vi "Store Configuration Parameters.vi"(8 "error in (no error)":errorcluster, 10 "refnum":T1, 11 "Example Configuration Dialog in":refnum<class "Server Config.lvclass">) -> (0 "error out":errorcluster, 2 "refnum out":T1, 3 "Example Configuration Dialog out":refnum<class "Server Config.lvclass">)   [LabVIEW 2016, in "Server Controller.lvlib" / "Server Config.lvclass"]
uses:
  Server Config.lvclass
  <vilib>/Utility/config.llb/Config Data RefNum.ctl
  Server Config.lvclass/Server Config.ctl
  MAL-Framework/user.lib/Common Components/Msmt Configuration/Controller Configuration.lvclass
  <vilib>/Utility/config.llb/NI_LVConfig.lvlib
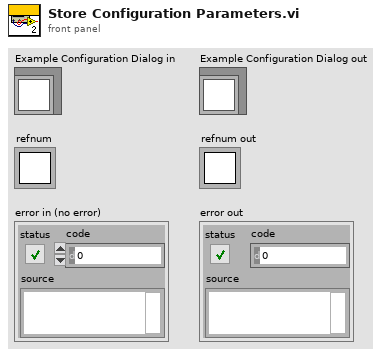
[diagram p1: front panel]
types:
  T1 = typedef "NI_LVConfig.lvlib/Config Data RefNum.ctl" = refnum<k1>
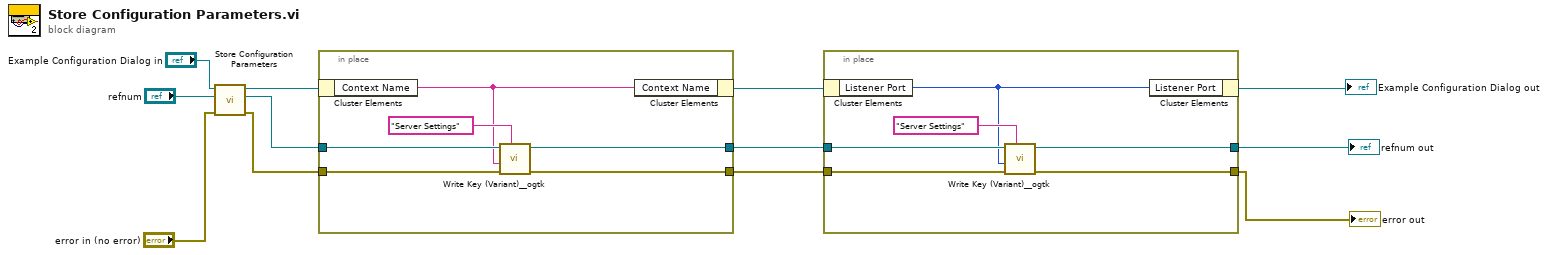
[diagram p0: block diagram]
diagram:
  n1 = call-parent "Store Configuration Parameters.vi"("error in (no error)"="error in (no error)", "refnum"="refnum", "Example Configuration Dialog in"="Example Configuration Dialog in") -> ("error out"=w7:errorcluster, "refnum out"=w8:T1, "Example Configuration Dialog out"=w9:refnum<class "Server Config.lvclass">)  [unwired: 6 in]
  n2 = in-place {
    in-place-border: w8 -> [w18]
    in-place-border: [w17] -> w5
    in-place-border: [w16] -> w4
    in-place-border: w7 -> [w13]
    n3 = in-place-cluster #1(w9) -> ("Context Name"=w14:string)
    n4 = call <userlib>:"Write Key (Variant)__ogtk.vi"("section"="Server Settings", "error in (no error)"=w13, "key-value"=w14, "refnum"=w18) -> ("error out"=w16:errorcluster, "refnum out"=w17:T1)  [unwired: 6 in]
    n5 = in-place-cluster #1("Context Name"=w14) -> (w6:refnum<class "Server Config.lvclass">)
  }
  n6 = in-place {
    in-place-border: w5 -> [w24]
    in-place-border: [w23] -> w2
    in-place-border: [w22] -> w1
    in-place-border: w4 -> [w19]
    n7 = in-place-cluster #2(w6) -> ("Listener Port"=w20:u16)
    n8 = call <userlib>:"Write Key (Variant)__ogtk.vi"("section"="Server Settings", "error in (no error)"=w19, "key-value"=w20, "refnum"=w24) -> ("error out"=w22:errorcluster, "refnum out"=w23:T1)  [unwired: 6 in]
    n9 = in-place-cluster #2("Listener Port"=w20) -> (→"Example Configuration Dialog out":refnum<class "Server Config.lvclass">)
  }
  "error out" <- w1
  "refnum out" <- w2
